vi "BuildPrinterFolder.vi"() -> ()   [LabVIEW 2014]
panel:
  out "2D Picture":picture
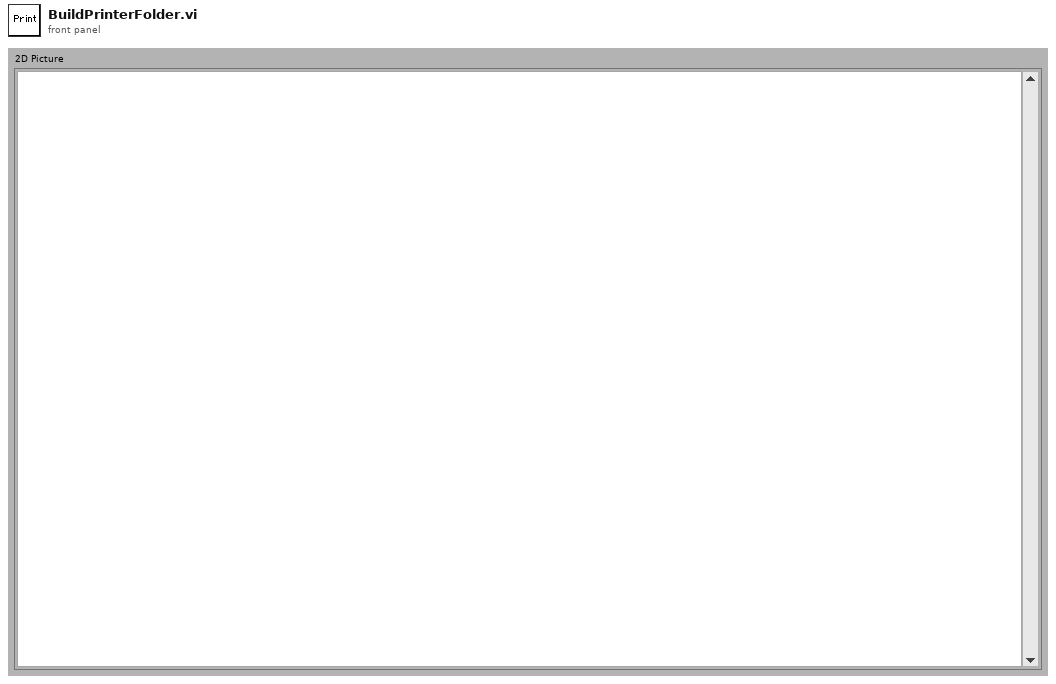
[diagram p1: front panel]
types:
  T1 = typedef "SlideTypeDef.ctl" = cluster{"Slide path":string, "Transition":enum16{"Pan", "Zoom-pan-zoom", "Zoom-wait-Zoom"}, "frame":cluster{"left":i16, "top":i16, "right":i16, "bottom":i16}, "Number":i32}
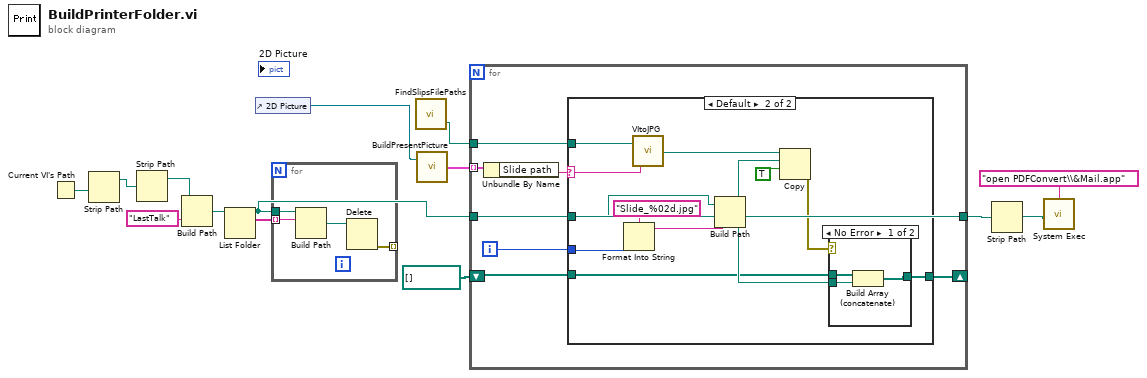
[diagram p0: block diagram]
diagram:
  n1 = Current VI's Path() -> (path=w8:path)
  n2 = Strip Path(path=w8) -> (stripped path=w9:path)  [unwired: 1 out]
  n3 = Strip Path(path=w9) -> (stripped path=w4:path)  [unwired: 1 out]
  n4 = Build Path(base path=w4, name or relative path="LastTalk") -> (appended path=w6:path)
  n5 = List Folder(path=w6) -> (path out=w1:path, filenames=w5:string[])  [unwired: 3 in, 2 out]
  n6 = control-ref of="2D Picture"() -> (w14:refnum<vi>)
  n7 = for {
    tunnel: w1 -> [w15]
    tunnel: w5 -> [w18] mode=indexing
    tunnel: [w16] -> _ mode=indexing
    n8 = Build Path(base path=w15, name or relative path=w18) -> (appended path=w17:path)
    n9 = Delete(path (use dialog)=w17) -> (error out=w16:errorcluster)  [unwired: 4 in, 2 out]
  }
  n10 = call "FindSlipsFilePaths.vi"() -> ("Images"=w12:path)  [unwired: 2 in, 4 out]
  n11 = call "BuildPresentPicture.vi"("Pict Refnum"=w14) -> ("SlideInfo"=w13:T1[])  [unwired: 2 in, 1 out]
  n12 = for {
    tunnel: w13 -> [w25] mode=indexing
    tunnel: w12 -> [w23]
    tunnel: w1 -> [w19]
    shift-right: [w21] -> _
    shift-left: path[] [] -> [w20]
    tunnel: [w19] -> w3
    i -> [w22]
    n13 = Unbundle By Name(w25) -> ("Slide path"=w24:string)
    n14 = case shown="Default" w24 {
      selector: w24 -> [_ w34]
      tunnel: w23 -> [_ w33]
      tunnel: w22 -> [_ w38]
      tunnel: w19 -> [_ w35]
      tunnel: [w26 w29] -> w21
      tunnel: w20 -> [w26 w28]
      frame "" {
      }
      frame Default {
        n15 = Format Into String(format string="Slide_%02d.jpg", w38) -> (resulting string=w36:string)  [unwired: 2 in, 1 out]
        n16 = call "VItoJPG.vi"("name"=w34, "Dest"=w33) -> ("appended path"=w32:path)
        n17 = Build Path(base path=w35, name or relative path=w36) -> (appended path=w30:path)
        n18 = Copy(9:TRUE ("overwrite (F)"), 10:w30, 11:w32) -> (0:w27:errorcluster)  [unwired: 2 in, 2 out]
        n19 = case shown="No Error" w27 {
          tunnel: w30 -> [w41 _]
          tunnel: [w40 w42] -> w29
          tunnel: w28 -> [w39 w42]
          frame No Error {
            n20 = Build Array (concatenate)(w39, w41) -> (w40:path[])
          }
          frame Error {
          }
        }
      }
    }
  }
  n21 = Strip Path(path=w3) -> (stripped path=w2:path)  [unwired: 1 out]
  n22 = call <vilib>:"System Exec.vi"("working directory"=w2, "command line"="open PDFConvert\\&Mail.app") -> ()  [unwired: 6 in, 4 out]
